vi "Only_Dashes.vi"(11 "Eingabetabelle":string[](array[string])) -> (3 "Dashes_only":bool)   [LabVIEW 2020, in "Linearisierung v2.lvlib" / "SpanEinstellungen.lvlib"]
uses:
  SpanEinstellungen.lvlib
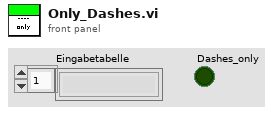
[diagram p1: front panel]
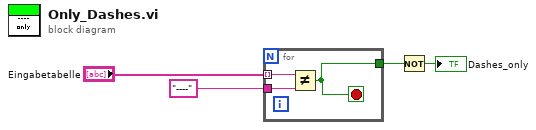
[diagram p0: block diagram]
diagram:
  n1 = for {
    tunnel: "Eingabetabelle" -> [w7] mode=indexing
    tunnel: "----" ("Nach String/Zeichen suchen (-)") -> [w6]
    tunnel: [w5] -> w2
    stop <- w5 stop-if-true
    n2 = Not Equal?(x=w7, y=w6) -> (x != y?=w5:bool)
  }
  n3 = Not(x=w2) -> (.not. x?=→"Dashes_only":bool)
